vi "Start trigger source handling.vi"(5 "sync.trigger":bool, 7 "trig.pxi trig src":i32, 9 "Refnum in":refnum<k21>, 12 "trig.source":T1) -> (4 "trigger":bool, 8 "aurora.data":u16, 10 "pxi.trig count":u16, 15 "aurora.trig count":u16)   [LabVIEW 2019, in "FPGA Utility.lvlib"]
doc: "Handles start trigger source. Several different sources are supported.\n\n<b>trig.source</b> - selects start trigger source, supported values: Use Tclk, PXI trigger and Aurora trigger"
uses:
  FPGA Utility.lvlib
  FPGA driver trigger source.ctl
  <vilib>/rvi/eio/common/nirviEmuTemplateMethod_errors.vi
  <instrlib>/_niInstr/Basic Elements/v1/FPGA/Private/Count Up U16.vi
  <vilib>/eio/EIONode/EIONode.xnode
  <vilib>/eio/EIOMethodNode/EIOMethodNode.xnode
  <instrlib>/_niInstr/Basic Elements/v1/FPGA/niInstr Basic Elements v1 FPGA.lvlib
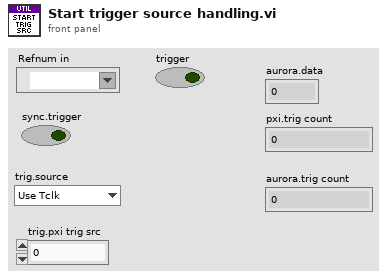
[diagram p1: front panel]
types:
  T1 = typedef "FPGA Utility.lvlib/FPGA driver trigger source.ctl" = enum16{"Use Tclk", "PXI_Trig", "Aurora RX trig"}
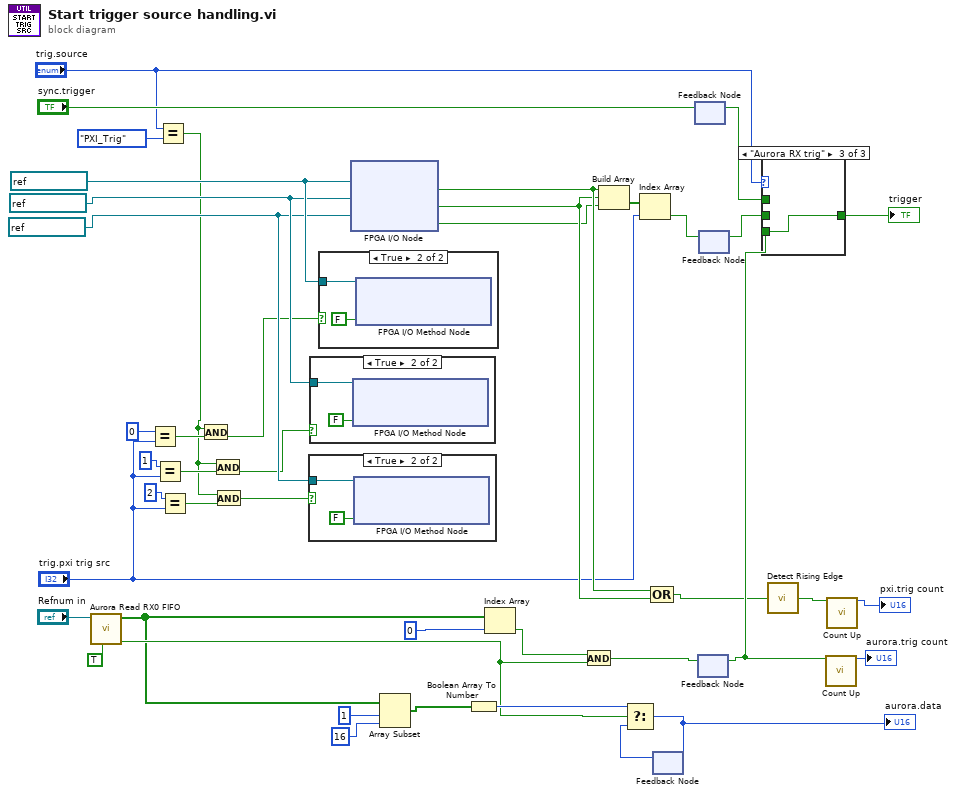
[diagram p0: block diagram]
diagram:
  w9 = refnum<k21> "PXI_Trig2" ("FPGA I/O In")
  w16 = refnum<k21> "PXI_Trig1" ("FPGA I/O In")
  w18 = refnum<k21> "PXI_Trig0" ("FPGA I/O In")
  n1 = call "Aurora Read RX0 FIFO.vi"("Ready for Output (T)"=TRUE, "Aurora FIFO"="Refnum in") -> ("Output Valid"=w40:bool, "Data"=w33:bool[])  [unwired: 8 in]
  n2 = Equal?(x=0, y="trig.pxi trig src") -> (x = y?=w15:bool)
  n3 = Equal?(x=1, y="trig.pxi trig src") -> (x = y?=w12:bool)
  n4 = Equal?(x="trig.source", y=FPGA_driver_trigger_source."PXI_Trig") -> (x = y?=w3:bool)
  n5 = Equal?(x=2, y="trig.pxi trig src") -> (x = y?=w4:bool)
  n6 = And(x=w3, y=w15) -> (x .and. y?=w8:bool)
  n7 = And(x=w3, y=w12) -> (x .and. y?=w5:bool)
  n8 = And(x=w3, y=w4) -> (x .and. y?=w2:bool)
  n9 = case shown="True" w2 {
    tunnel: w9 -> [_ w45]
    frame False {
    }
    frame True {
      n10 = xnode "FPGA I/O Method Node"("FPGA I/O In"=w45, "Enable"=FALSE ("Data")) -> ()  [unwired: 1 out]
    }
  }
  n11 = case shown="True" w5 {
    tunnel: w16 -> [_ w47]
    frame False {
    }
    frame True {
      n12 = xnode "FPGA I/O Method Node"("FPGA I/O In"=w47, "Enable"=FALSE ("Data")) -> ()  [unwired: 1 out]
    }
  }
  n13 = case shown="True" w8 {
    tunnel: w18 -> [_ w49]
    frame False {
    }
    frame True {
      n14 = xnode "FPGA I/O Method Node"("FPGA I/O In"=w49, "Enable"=FALSE ("Data")) -> ()  [unwired: 1 out]
    }
  }
  n15 = xnode "FPGA I/O Node"("FPGA I/O In"=w18, "FPGA I/O In"=w16, "FPGA I/O In"=w9) -> ("I/O Item"=w21:bool, "I/O Item"=w20:bool, "I/O Item"=w10:bool)  [unwired: 3 out]
  n16 = Array Subset(array=w33, index=1, length=16 ("index")) -> (w36:bool[])
  n17 = Boolean Array To Number(Boolean array=w36) -> (number=w41:u16)
  n18 = Index Array(array=w33, index=0) -> (element=w32:bool)
  n19 = And(x=w32, y=w40) -> (x .and. y?=w27:bool)
  n20 = Build Array(w21, w20, w10) -> (w29:bool[])
  n21 = Index Array(array=w29, index="trig.pxi trig src") -> (element=w30:bool)
  n22 = Compound Arithmetic op=OR(w21, w20) -> (w19:bool)
  n23 = feedback #1() -> (w42:u16)  [unwired: 1 in]
  n24 = Select(t=w41, s=w40, f=w42) -> (s? t:f=w43:u16)
  "aurora.data" <- w43
  n25 = feedback-in #1(w43) -> ()
  n26 = feedback #2() -> (w24:bool)  [unwired: 1 in]
  n27 = feedback-in #2("sync.trigger") -> ()
  n28 = feedback #3() -> (w26:bool)  [unwired: 1 in]
  n29 = feedback-in #3(w27) -> ()
  n30 = feedback-in #4(w30) -> ()
  n31 = feedback #4() -> (w23:bool)  [unwired: 1 in]
  n32 = case shown="\"Aurora RX trig\"" "trig.source" {
    tunnel: w24 -> [w50 _ _]
    tunnel: [w50 w51 w52] -> w39
    tunnel: w23 -> [_ w51 _]
    tunnel: w26 -> [_ _ w52]
    frame "Use Tclk", Default {
    }
    frame "PXI_Trig" {
    }
    frame "Aurora RX trig" {
    }
  }
  "trigger" <- w39
  n33 = call <instrlib>:"Detect Rising Edge.vi"("signal"=w19) -> ("edge detected"=w1:bool)  [unwired: 14 in]
  n34 = call-poly <instrlib>:"Count Up.vi"("increment"=w26) -> ("count out"=→"aurora.trig count":u16)  [unwired: 14 in]
  n35 = call-poly <instrlib>:"Count Up.vi"("increment"=w1) -> ("count out"=→"pxi.trig count":u16)  [unwired: 14 in]
